vi "Remove Item From Group.vi"(8 "error in (no error)":errorcluster, 11 "Selector in":refnum<class "Selector.lvclass">) -> (0 "error out":errorcluster, 3 "Selector out":refnum<class "Selector.lvclass">)   [LabVIEW 2019, in "Selector.lvclass"]
uses:
  Selector.lvclass
  Selector.lvclass/Selector.ctl
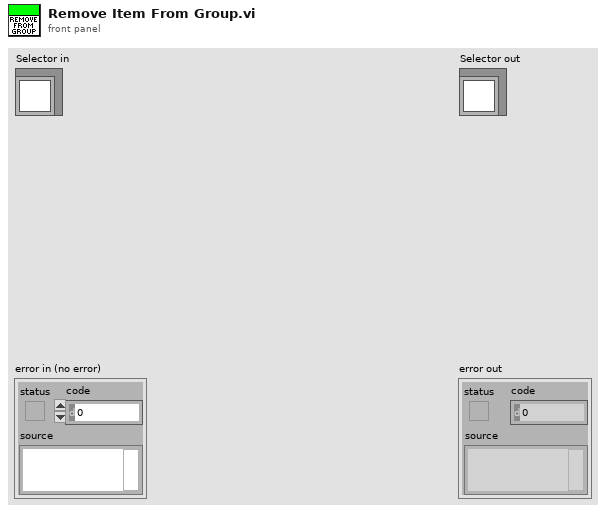
[diagram p1: front panel]
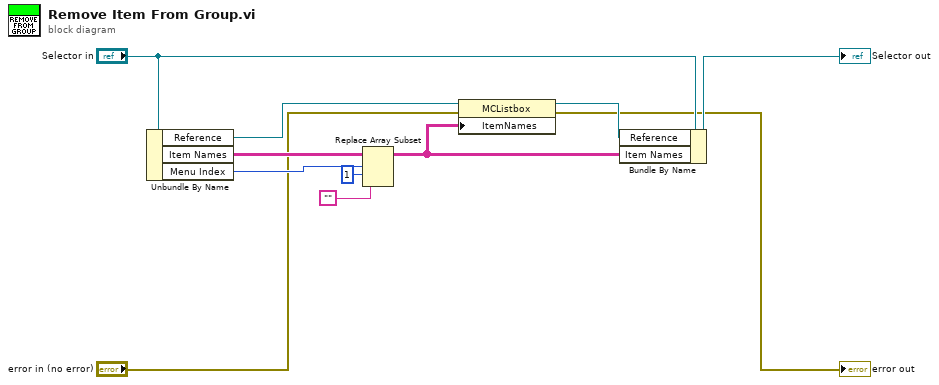
[diagram p0: block diagram]
diagram:
  n1 = Unbundle By Name("Selector in") -> ("Reference"=w6:refnum<vi>, "Item Names"=w5:string[][], "Menu Index"=w11:i32)
  n2 = Replace Array Subset(array=w5, new element="", index (row)=w11, index (col)=1 ("disabled index (col)")) -> (w1:string[][])
  n3 = property class="MCListbox"(reference=w6, error in="error in (no error)", "ItemNames"=w1) -> (reference out=w4:refnum<vi>, error out=→"error out":errorcluster)
  n4 = Bundle By Name(cluster="Selector in", "Reference"=w4, "Item Names"=w1) -> (→"Selector out":refnum<class "Selector.lvclass">)
